vi "Actor Core.vi"(8 "error in":errorcluster, 11 "Print View in":refnum<class "Print View.lvclass">) -> (0 "error out":errorcluster, 3 "Actor out":refnum<class "Actor.lvclass">)   [LabVIEW 2015, in "Print View.lvlib" / "Print View.lvclass"]
doc: "(<B>Filename</B>: Actor Framework.lvlib:Actor.lvclass:Actor Core.vi)\n\nReceives messages to the actor, reacts to them, and initiates any error handling that may shut the actor down.\n\nDescendant classes may override this VI to append parallel tasks for the actor to complete while it handles messages. Overrides use the Call Parent Method node."
uses:
  Print View.lvclass
  <vilib>/ActorFramework/Actor/Actor.lvclass
  <vilib>/ActorFramework/Actor/Actor.lvclass/Actor.ctl
  <vilib>/ActorFramework/Message Enqueuer/Message Enqueuer.lvclass/Message Enqueuer.ctl
  Print View Messages/Broadcast Print Msg/Broadcast Print Msg.lvclass/Broadcast Print Msg.ctl
  Print View Messages/Broadcast Cancel Msg/Broadcast Cancel Msg.lvclass/Broadcast Cancel Msg.ctl
  <vilib>/ActorFramework/Message Enqueuer/Init from Existing Queue.vi
  <vilib>/ActorFramework/Message Enqueuer/Enqueue.vi
  <vilib>/ActorFramework/Message Priority Queue/Priority Enqueue.vi
  <vilib>/ActorFrameworkMVC/Abstract View/Abstract View/Abstract View.lvclass
  <vilib>/ActorFramework/Message Enqueuer/Message Enqueuer.lvclass
  Print View Messages/Broadcast Print Msg/Broadcast Print Msg.lvclass
  Print View Messages/Broadcast Cancel Msg/Broadcast Cancel Msg.lvclass
panel:
  in  "Coppies Numeric Text Box":dbl=1.0
  in  "Pages String Text Box":string
  in  "Pages Radio Buttons":enum32{"All Radio Button", "Pages Radio Button"}(radio)
  in  "Change Printer Push Button":bool
  out "Printer Name":string="MiWiFi-R2D-SRV (HP Deskject 3540)"
  in  "Cancel Print Push Button":bool
  in  "Print Push Button":bool
  # "Destination"
  # "Pages"
  # "Copies"
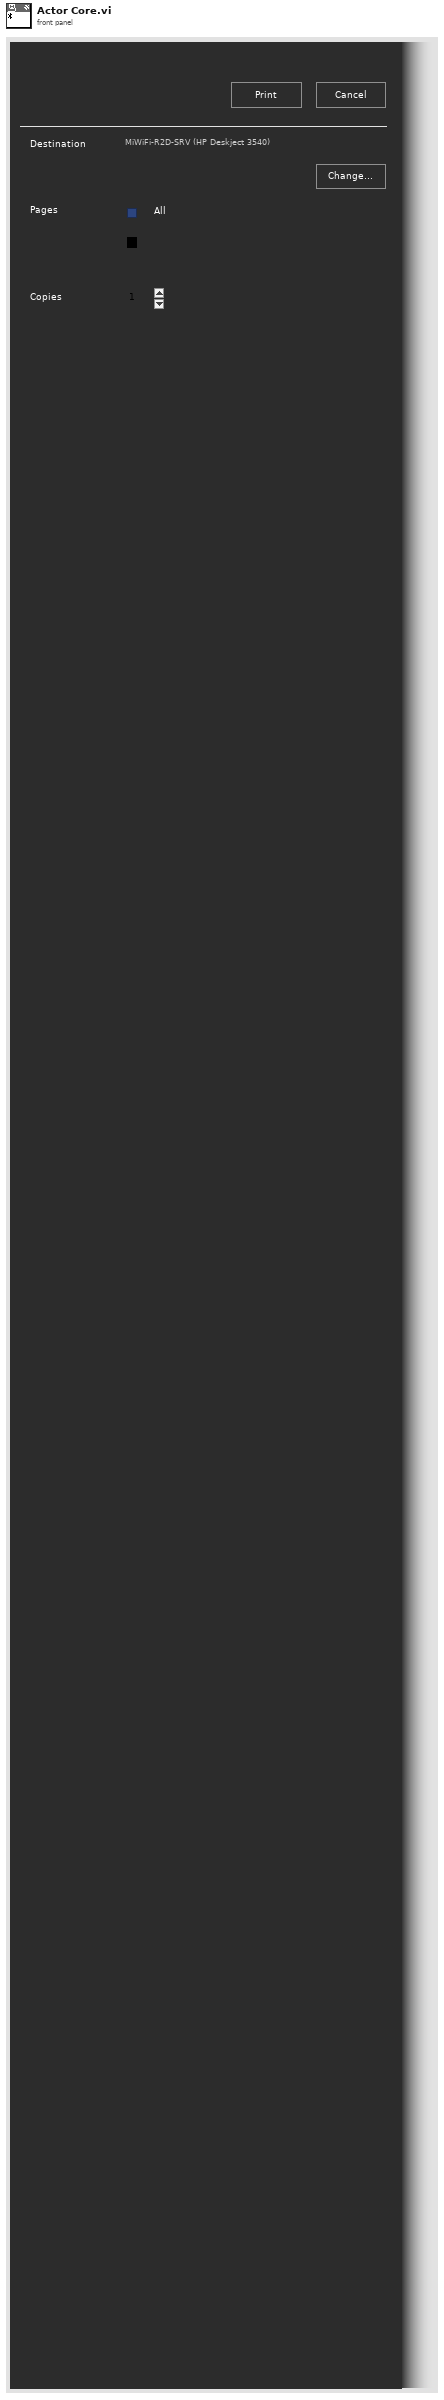
[diagram p1: front panel]
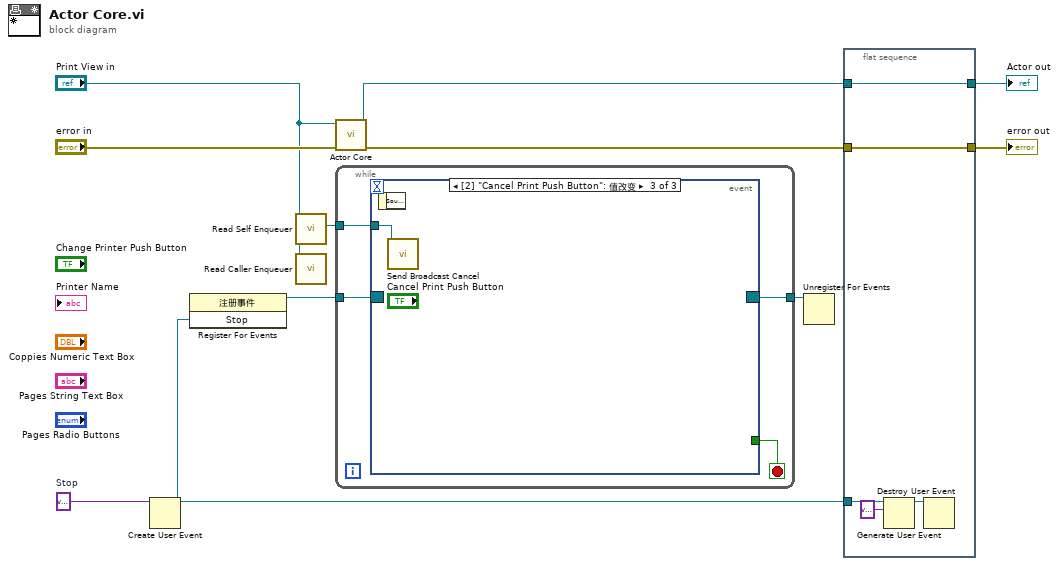
[diagram p0: block diagram]
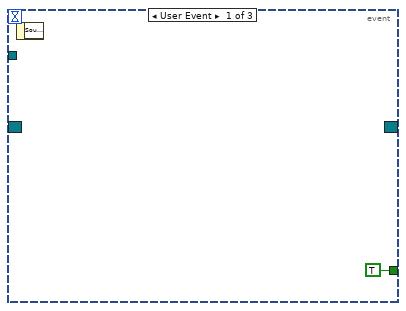
[diagram p2: hidden frame]
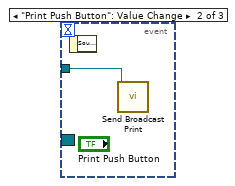
[diagram p3: hidden frame]
diagram:
  w9 = variant  # Stop
  n1 = Create User Event(user event datatype=w9) -> (user event=w5:refnum<user-event>)  [unwired: 1 in, 1 out]
  n2 = register-events(w5) -> (reference out=w10:refnum<event-registration>)  [unwired: 2 in, 1 out]
  n3 = call <vilib>:"Read Self Enqueuer.vi"("Actor"="Print View in") -> ("Self Enqueuer"=w11:refnum<class "Message Enqueuer.lvclass">)  [unwired: 10 in]
  n4 = call <vilib>:"Read Caller Enqueuer.vi"("Actor"="Print View in") -> ()  [unwired: 10 in, 1 out]
  n5 = call-parent "Actor Core.vi"("error in"="error in", "Abstract View in"="Print View in") -> ("error out"=w6:errorcluster, "Actor out"=w7:refnum<class "Actor.lvclass">)  [unwired: 8 in]
  n6 = while {
    tunnel: w11 -> [w12]
    tunnel: w10 -> [w15]
    tunnel: [w14] -> w8
    stop <- w13 stop-if-true
    n7 = event shown="[2] \"Cancel Print Push Button\": 值改变" {
      selector: w15 -> [_ _ _]
      dyn-events: [_ _ _] -> w14
      timeout: _ -> [_ _ _]
      tunnel: [TRUE _ _] -> w13
      tunnel: w12 -> [_ w17 w18]
      event User Event {
        n8 = event-data() -> ()  [unwired: 1 in, 1 out]
      }
      event "Print Push Button": Value Change {
        n9 = event-data() -> ()  [unwired: 1 in, 1 out]
        n10 = call "Send Broadcast Print.vi"("Message Enqueuer"=w17) -> ()  [unwired: 9 in, 2 out]
      }
      event "Cancel Print Push Button": Value Change {
        n11 = event-data() -> ()  [unwired: 1 in, 1 out]
        n12 = call "Send Broadcast Cancel.vi"("Message Enqueuer"=w18) -> ()  [unwired: 9 in, 2 out]
      }
    }
  }
  n13 = Unregister For Events(event registration refnum=w8) -> ()  [unwired: 1 in, 1 out]
  n14 = flat-sequence {
    tunnel: w5 -> [w23]
    tunnel: w7 -> [w20]
    tunnel: [w20] -> w3
    tunnel: w6 -> [w19]
    tunnel: [w19] -> w2
    frame #0 {
      n15 = Generate User Event(user event=w23, event data cluster=variant ("event data")) -> (user event out=w21:refnum<user-event>)  [unwired: 2 in, 1 out]
      n16 = Destroy User Event(user event=w21) -> ()  [unwired: 1 in, 1 out]
    }
  }
  "error out" <- w2
  "Actor out" <- w3
